vi "writeModbusTxData2.vi"(8 "error in (no error)":errorcluster, 9 "Timeout (ms)":i32, 10 "ModbusBuffer in":refnum<class "ModbusBuffer.lvclass">, 11 "FPGA in":refnum<class "FPGA.lvclass">) -> (0 "error out":errorcluster, 1 "Empty Elements Remaining":u32, 3 "FPGA out":refnum<class "FPGA.lvclass">)   [LabVIEW 2016, in "FPGA.lvclass"]
uses:
  FPGA.lvclass
  Common_RT_Modbus/ModbusBuffer/ModbusBuffer.lvclass
  FPGA.lvclass/FPGA.ctl
  Common_RT_Modbus/ModbusBuffer/ModbusBuffer.lvclass/ModbusBuffer.ctl
  <vilib>/Utility/error.llb/Error Cluster From Error Code.vi
  <vilib>/rvi/errors/niLvFpgaAdjustHostInterfaceError.vi
  <vilib>/rvi/interface/nirviMethod/nirviMethod.xnode
  <vilib>/FPGAPlugInAG/Dynamic/niLvFpga_WriteFifo_Dynamic.vi
  <vilib>/rvi/errors/niLvFpgaMergeErrorWithErrorCode.vi
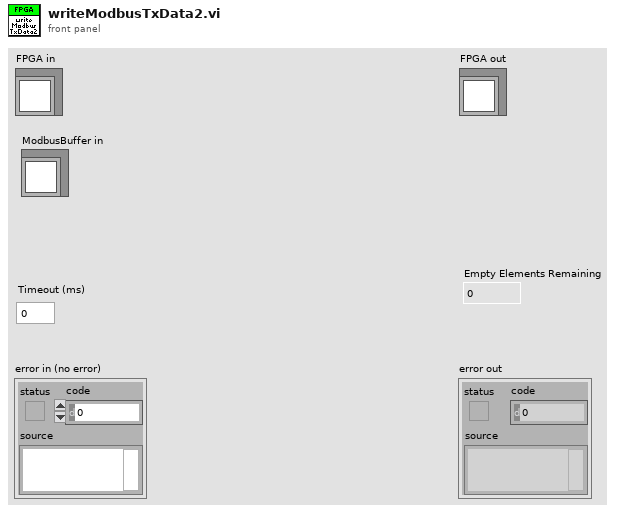
[diagram p1: front panel]
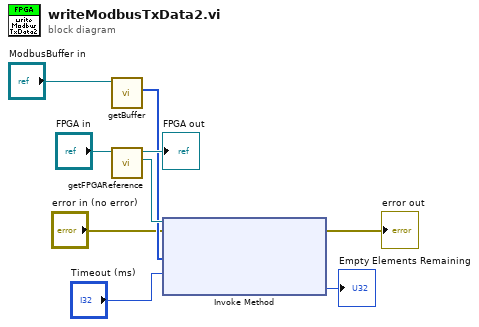
[diagram p0: block diagram]
diagram:
  n1 = call "getBuffer.vi"("ModbusBuffer in"="ModbusBuffer in") -> ("Buffer"=w3:u16[])  [unwired: 9 in, 1 out]
  n2 = call "getFPGAReference.vi"("FPGA in"="FPGA in") -> ("FPGAReference"=w8:refnum<k20>, "FPGA out"=→"FPGA out":refnum<class "FPGA.lvclass">)  [unwired: 9 in]
  n3 = xnode "Invoke Method"("FPGA VI Reference In"=w8, "error in"="error in (no error)", "Data"=w3, "Timeout (ms)"="Timeout (ms)") -> ("error out"=→"error out":errorcluster, "Empty Elements Remaining"=→"Empty Elements Remaining":u32)  [unwired: 1 out]
